vi "DB_Delete Data.vi"(7 "condition":string, 8 "error in (no error)":errorcluster, 10 "table":string, 11 "connection reference":T1) -> (0 "error out":errorcluster)   [LabVIEW 2017]
uses:
  <vilib>/addons/database/Connection.llb/Conn ObjectReference.ctl
  <vilib>/addons/database/NI_Database_API.lvlib
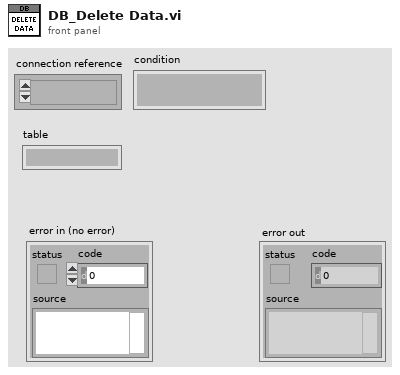
[diagram p1: front panel]
types:
  T1 = typedef "NI_Database_API.lvlib/Conn ObjectReference.ctl" = refnum<k1>
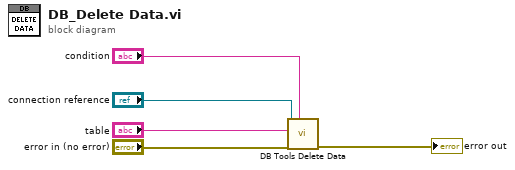
[diagram p0: block diagram]
diagram:
  n1 = call <vilib>:"DB Tools Delete Data.vi"("condition"="condition", "error in (no error)"="error in (no error)", "table"="table", "connection reference"="connection reference") -> ("error out"=→"error out":errorcluster)  [unwired: 6 in, 1 out]
